vi "RAMP_single_scan.vi"(4 "Pulse length Ton (s)":dbl=0.009999999776482582, 6 "queue CAMERA":refnum<queue>, 7 "queue piezo":refnum<queue>, 8 "error in":errorcluster, 9 "Illumination source":bool, 10 "N laser lines":i32, 11 "Ramp":dbl[](array[numeric])) -> (0 "error out":errorcluster)   [LabVIEW 2015]
uses:
  CONTROLS/Q_MCL_piezo_element.ctl
  CONTROLS/Q_camera_element.ctl
  GLOBAL/Global_ABORT.vi
  GLOBAL/Global_MAIN.vi
  GLOBAL/Global_CAMERA.vi
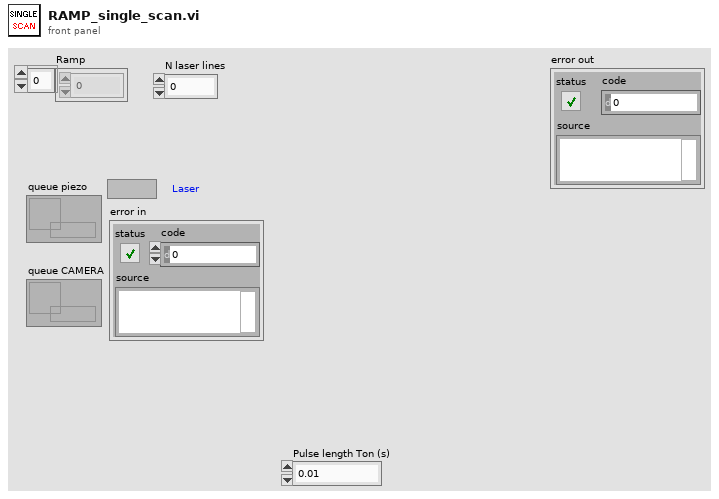
[diagram p1: front panel]
types:
  T1 = typedef "Q_MCL_piezo_element.ctl" = cluster{"variant":variant, "Instruction":enum16{"Piezo_idle", "Piezo_initialize", "Piezo_error", "Piezo_security_stop", "Piezo_read_z", "Piezo_move_z", "Piezo_keyboard_move", "Piezo_close_autofocus_calibration_ramp", "Piezo_change_init_state", "Piezo_init_autofocus", "Piezo_init_autofocus_merFISH_TL", "Piezo_autofocus", "Piezo_autofocus_merFISH_TL", "Piezo_stop_autofocus", "Piezo_stop_autofocus_merFISH_TL", "Piezo_autofocus_lost", "Piezo_resume_autofocus_merFISH_TL", "Piezo_check_z_position_merFISH_TL", "Piezo_init_ramp", "Piezo_move_z_ramp", "Piezo_close_ramp", "Piezo_close_merFISH", "Piezo_stop"}}
  T2 = cluster{"Pulse length Ton (s)":dbl, "image #":i32, "Display?":bool}
  T3 = typedef "Q_camera_element.ctl" = cluster{"variant":variant, "Instruction":enum16{"CAMERA_idle", "CAMERA_initialize", "CAMERA_error", "CAMERA_security_stop", "CAMERA_not_acquiring", "CAMERA_acquiring", "CAMERA_start_acquiring", "CAMERA_stop_acquiring", "CAMERA_change_exposure", "CAMERA_define_ROI", "CAMERA_cooler", "CAMERA_acquire_movie", "CAMERA_init_scan", "CAMERA_check_new_scan_image", "CAMERA_close_scan", "CAMERA_init_merFISH", "CAMERA_start_acquiring_merFISH", "CAMERA_close_scan_merFISH", "CAMERA_close_merFISH", "CAMERA_init_TL", "CAMERA_start_acquiring_TL", "CAMERA_stop_acquiring_TL", "CAMERA_close_TL", "CAMERA_STOP"}}
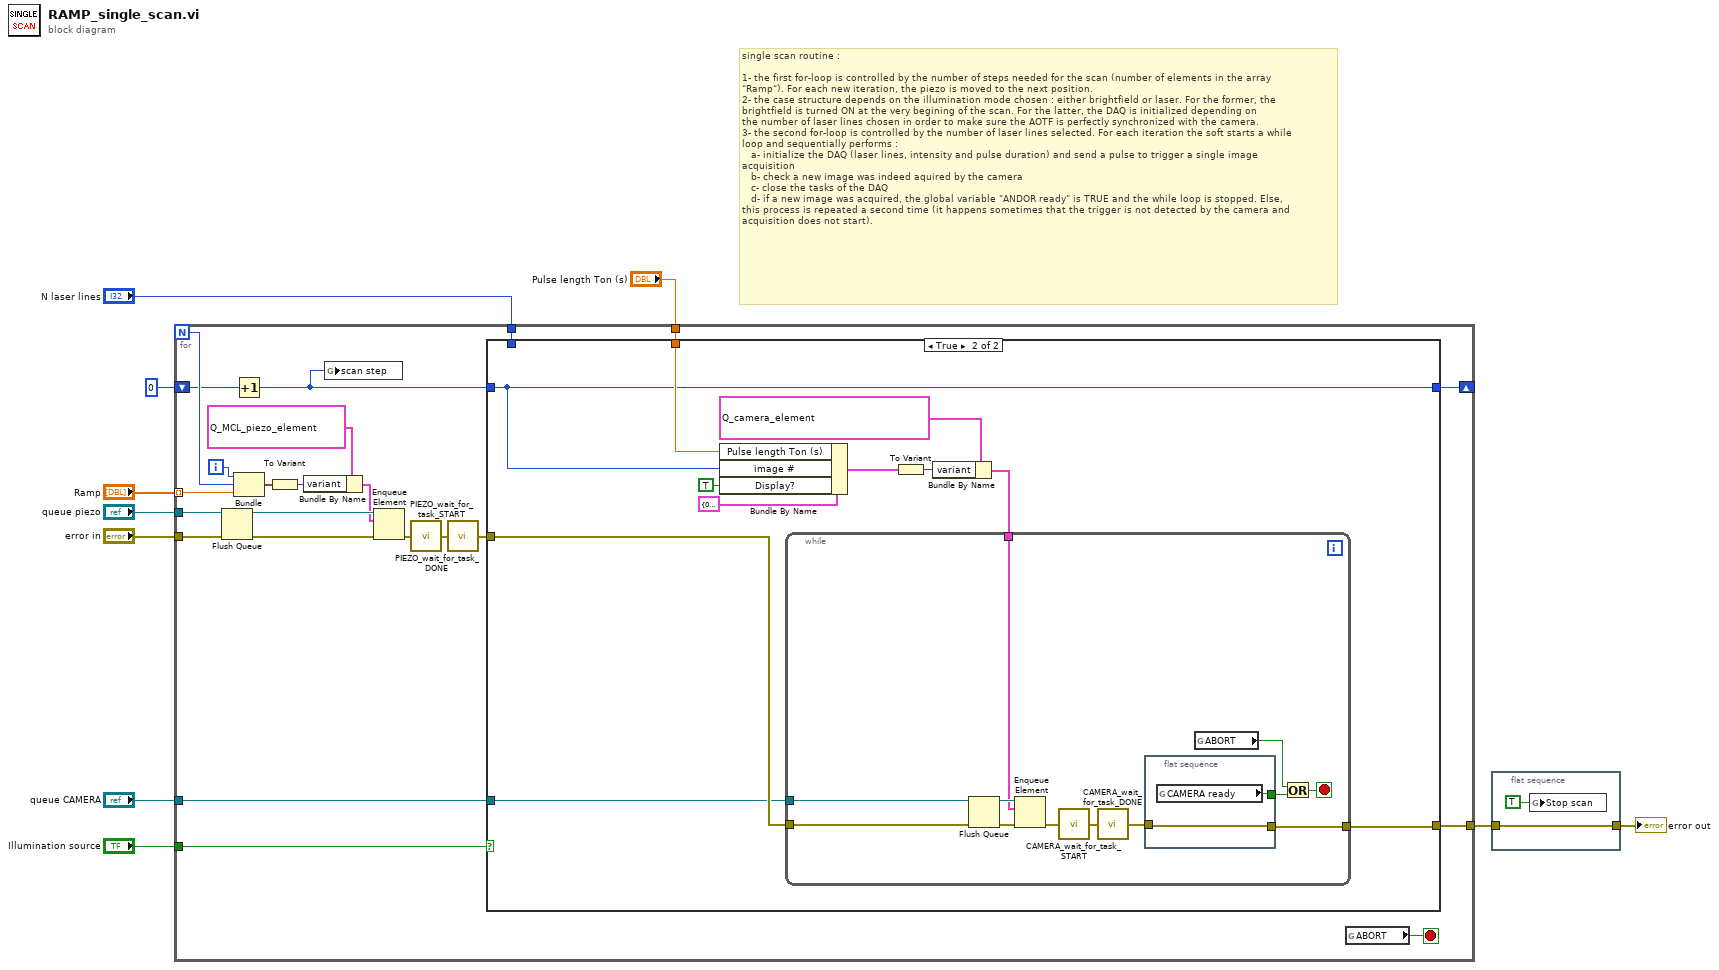
[diagram p0: block diagram]
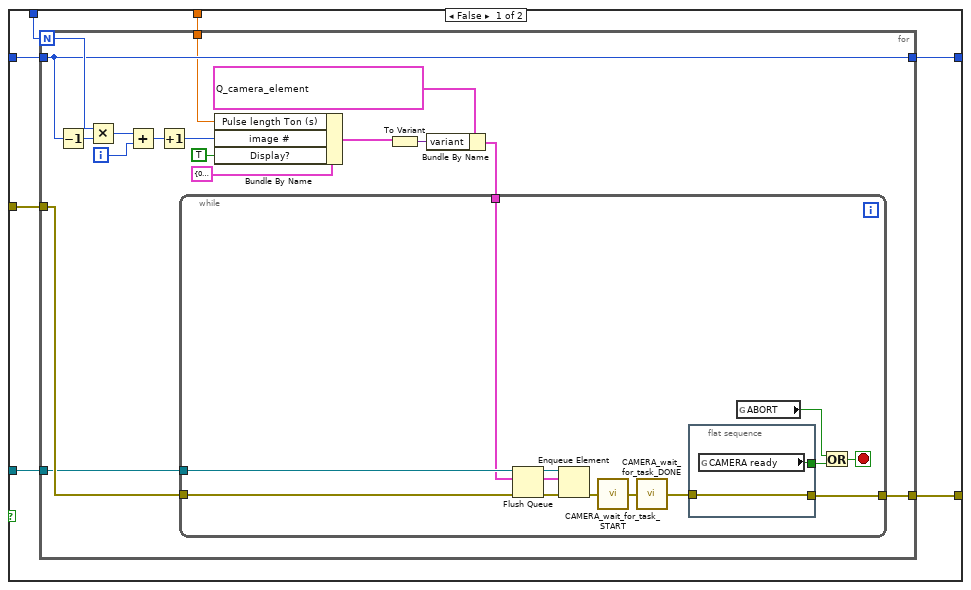
[diagram p2: hidden frame]
diagram:
  # "single scan routine :\n\n1- the first for-loop is controlled by the number of steps needed for the scan (number of elements in the array\n\"Ramp\"). For each new iteration, the piezo is moved to the next position.\n2- the case structure depends on the illumination mode chosen : either brightfield or laser. For the former, the\nbrightfield is turned ON at the very begining of the scan. For the latter, the DAQ is initialized depending on\nthe number of laser lines chosen in order to make sure the AOTF is perfectly synchronized with the camera.\n3- the second for-loop is controlled by the number of laser lines selected. For each iteration the soft starts a while\nloop and sequentially performs :\n   a- initialize the DAQ (laser lines, intensity and pulse duration) and send a pulse to trigger a single image\nacquisition\n   b- check a new image was indeed aquired by the camera\n   c- close the tasks of the DAQ\n   d- if a new image was acquired, the global variable \"ANDOR ready\" is TRUE and the while loop is stopped. Else, \nthis process is repeated a second time (it happens sometimes that the trigger is not detected by the camera and\nacquisition does not start)."
  n1 = for {
    N -> [w16]
    tunnel: "Ramp" -> [w18] mode=indexing
    tunnel: "queue piezo" -> [w33]
    shift-right: [w13] -> _
    shift-left: 0 -> [w14]
    tunnel: "queue CAMERA" -> [w24]
    tunnel: "Pulse length Ton (s)" -> [w23]
    tunnel: [w22] -> w2
    tunnel: "Illumination source" -> [w15]
    tunnel: "error in" -> [w20]
    tunnel: "N laser lines" -> [w11]
    i -> [w17]
    stop <- w21 stop-if-true
    n2 = Flush Queue(queue=w33, error in (no error)=w20) -> (queue out=w30:refnum<queue>, error out=w29:errorcluster)  [unwired: 1 out]
    n3 = Increment(x=w14) -> (x+1=w12:i32)
    n4 = Bundle(w17, w16, w18) -> (w19:cluster{i32, i32, dbl})  [unwired: 1 in]
    n5 = To Variant(anything=w19) -> (Variant=w31:variant)
    n6 = Bundle By Name(cluster=T1 {"variant"=variant, "Instruction"=enum."Piezo_move_z_ramp"} ("Q_MCL_Piezo"), "variant"=w31) -> (w28:T1)
    n7 = global write "Global_MAIN.vi" "scan step"(w12) -> ()
    n8 = Enqueue Element(queue=w30, element=w28, error in (no error)=w29) -> (error out=w27:errorcluster)  [unwired: 1 in, 2 out]
    n9 = call "PIEZO_wait_for_task_START.vi"("error in"=w27) -> ("error out"=w26:errorcluster)
    n10 = call "PIEZO_wait_for_task_DONE.vi"("error in"=w26) -> ("error out"=w25:errorcluster)
    n11 = case shown="True" w15 {
      tunnel: w25 -> [w40 w82]
      tunnel: [w39 w73] -> w13
      tunnel: w24 -> [w38 w78]
      tunnel: w23 -> [w37 w74]
      tunnel: [w36 w77] -> w22
      tunnel: w12 -> [w35 w73]
      tunnel: w11 -> [w34 _]
      frame False {
        n12 = for {
          N: w34 -> [w56]
          tunnel: w40 -> [w57]
          tunnel: [w55] -> w39
          tunnel: w35 -> [w55]
          tunnel: w38 -> [w51]
          tunnel: w37 -> [w42]
          tunnel: [w47] -> w36
          i -> [w53]
          n13 = Decrement(x=w55) -> (x-1=w46:i32)
          n14 = Multiply(x=w56, y=w46) -> (x*y=w54:i32)
          n15 = Add(x=w54, y=w53) -> (x+y=w52:i32)
          n16 = Increment(x=w52) -> (x+1=w41:i32)
          n17 = Bundle By Name(cluster=T2 {"Pulse length Ton (s)"=0.0, "image #"=0, "Display?"=FALSE} ("output cluster"), "Pulse length Ton (s)"=w42, "image #"=w41, "Display?"=TRUE) -> (w44:T2)
          n18 = To Variant(anything=w44) -> (Variant=w49:variant)
          n19 = Bundle By Name(cluster=T3 {"variant"=variant, "Instruction"=enum."CAMERA_check_new_scan_image"} ("Q_ANDOR_element"), "variant"=w49) -> (w48:T3)
          n20 = while {
            tunnel: w57 -> [w58]
            tunnel: w51 -> [w69]
            tunnel: w48 -> [w68]
            tunnel: [w67] -> w47
            stop <- w66 stop-if-true
            n21 = Flush Queue(queue=w69, error in (no error)=w58) -> (queue out=w63:refnum<queue>, error out=w62:errorcluster)  [unwired: 1 out]
            n22 = Enqueue Element(queue=w63, element=w68, error in (no error)=w62) -> (error out=w61:errorcluster)  [unwired: 1 in, 2 out]
            n23 = call "CAMERA_wait_for_task_START.vi"("error in"=w61) -> ("error out"=w60:errorcluster)
            n24 = call "CAMERA_wait_for_task_DONE.vi"("error in"=w60) -> ("error out"=w59:errorcluster)
            n25 = flat-sequence {
              tunnel: [w70] -> w65
              tunnel: [w71] -> w67
              tunnel: w59 -> [w71]
              frame #0 {
                n26 = global read "Global_CAMERA.vi" "CAMERA ready"() -> (w70:bool)
              }
            }
            n27 = global read "Global_ABORT.vi" "ABORT"() -> (w64:bool)
            n28 = Or(x=w64, y=w65) -> (x .or. y?=w66:bool)
          }
        }
      }
      frame True {
        n29 = Bundle By Name(cluster=T2 {"Pulse length Ton (s)"=0.0, "image #"=0, "Display?"=FALSE} ("output cluster"), "Pulse length Ton (s)"=w74, "image #"=w73, "Display?"=TRUE) -> (w72:T2)
        n30 = To Variant(anything=w72) -> (Variant=w80:variant)
        n31 = Bundle By Name(cluster=T3 {"variant"=variant, "Instruction"=enum."CAMERA_check_new_scan_image"} ("Q_ANDOR_element"), "variant"=w80) -> (w79:T3)
        n32 = while {
          tunnel: [w94] -> w77
          tunnel: w82 -> [w83]
          tunnel: w79 -> [w84]
          tunnel: w78 -> [w86]
          stop <- w93 stop-if-true
          n33 = Flush Queue(queue=w86, error in (no error)=w83) -> (queue out=w87:refnum<queue>, error out=w88:errorcluster)  [unwired: 1 out]
          n34 = Enqueue Element(queue=w87, element=w84, error in (no error)=w88) -> (error out=w89:errorcluster)  [unwired: 1 in, 2 out]
          n35 = call "CAMERA_wait_for_task_START.vi"("error in"=w89) -> ("error out"=w90:errorcluster)
          n36 = call "CAMERA_wait_for_task_DONE.vi"("error in"=w90) -> ("error out"=w85:errorcluster)
          n37 = flat-sequence {
            tunnel: [w96] -> w92
            tunnel: [w95] -> w94
            tunnel: w85 -> [w95]
            frame #0 {
              n38 = global read "Global_CAMERA.vi" "CAMERA ready"() -> (w96:bool)
            }
          }
          n39 = global read "Global_ABORT.vi" "ABORT"() -> (w91:bool)
          n40 = Or(x=w91, y=w92) -> (x .or. y?=w93:bool)
        }
      }
    }
    n41 = global read "Global_ABORT.vi" "ABORT"() -> (w21:bool)
  }
  n42 = flat-sequence {
    tunnel: w2 -> [w97]
    tunnel: [w97] -> w3
    frame #0 {
      n43 = global write "Global_MAIN.vi" "Stop scan"(TRUE ("Stop scan")) -> ()
    }
  }
  "error out" <- w3
